vi "Retrieve Root Actor.vi"(8 "error in (no error)":errorcluster, 11 "INI Store in":refnum<class "INI Store.lvclass">) -> (0 "error out":errorcluster, 1 "valid?":bool, 2 "Root Actor":path, 3 "INI Store out":refnum<class "INI Store.lvclass">)   [LabVIEW 2023, in "Add Async Methods Actor.lvlib" / "INI Store.lvclass"]
uses:
  INI Store.lvclass
  <resource>/dialog/lvconfig.llb/LV Config Read Pathlist.vi
  INI Store.lvclass/INI Store.ctl
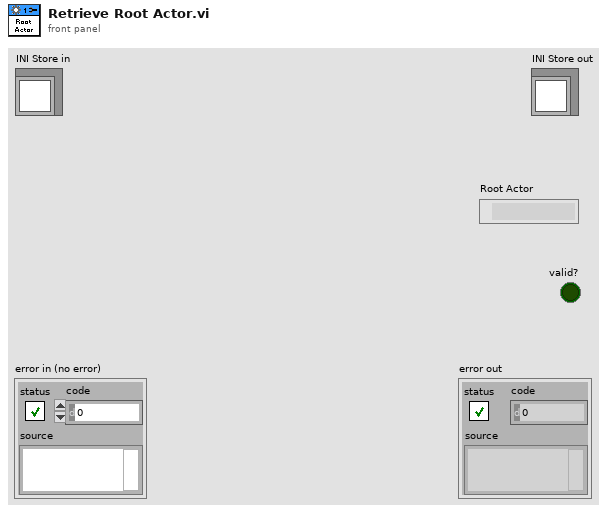
[diagram p1: front panel]
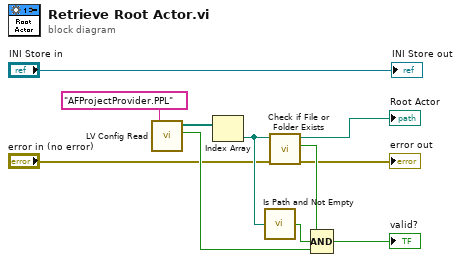
[diagram p0: block diagram]
diagram:
  n1 = call-poly <resource>:"LV Config Read.vi"("key"="AFProjectProvider.PPL") -> ("found?"=w9:bool, "value"=w11:path[])  [unwired: 4 in, 1 out]
  n2 = Index Array(array=w11) -> (element=w8:path)  [unwired: 1 in]
  n3 = call <vilib>:"Is Path and Not Empty.vi"("path"=w8) -> ("Is Path and Not Empty?"=w7:bool)  [unwired: 4 in]
  n4 = call <vilib>:"Check if File or Folder Exists.vi"("error in (no error)"="error in (no error)", "path"=w8) -> ("error out"=→"error out":errorcluster, "file or folder exists?"=w10:bool, "dup path"=→"Root Actor":path)  [unwired: 7 in]
  n5 = Compound Arithmetic op=AND(w10, w7, w9) -> (→"valid?":bool)
  "INI Store out" <- "INI Store in"
